vi "5.1-6.7.1-Act Client.vi"() -> ()   [LabVIEW 2010]
doc: "This VI implements a client for the Named Service UDP Server.vi.\nIt connects to a service by specifying the server address and the name of the service. After sending a 'Hello' string to the server, the client receives the string sent by the server, displays the string and closes the connection.\n\n<b>Note:</b> This VI is built to work with the Named Service UDP Server.vi in UDP.llb."
uses:
  6-OCU Neurons/MDF LatLong.ctl
  6-OCU Neurons/MDF Array LatLong.ctl
  6-OCU Neurons/6.1-UDP Saitek.ctl
  6-OCU Neurons/MainControls.ctl
  5.0-Global.vi
panel:
  out "data":T1 {"5.1.1 MDF GPS 2"."Latitude (waypoint)" format="%#_8g"; "5.1.1 MDF GPS 2"."Longitude  (waypoint)" format="%#_8g"; "6.1-Saitek Controller"."Right" scale=-32767.0..32767.0; "6.1-Saitek Controller"."Left" scale=-32767.0..32767.0; "6.1-Saitek Controller"."Yaw" scale=-32767.0..32767.0; "6.1-Saitek Controller"."Roll" scale=-32767.0..32767.0; "6.1-Saitek Controller"."Pitch" scale=-32767.0..32767.0}
  out "String":string
  out "error out":errorcluster
  in  "stop":bool
  in  "error in":errorcluster
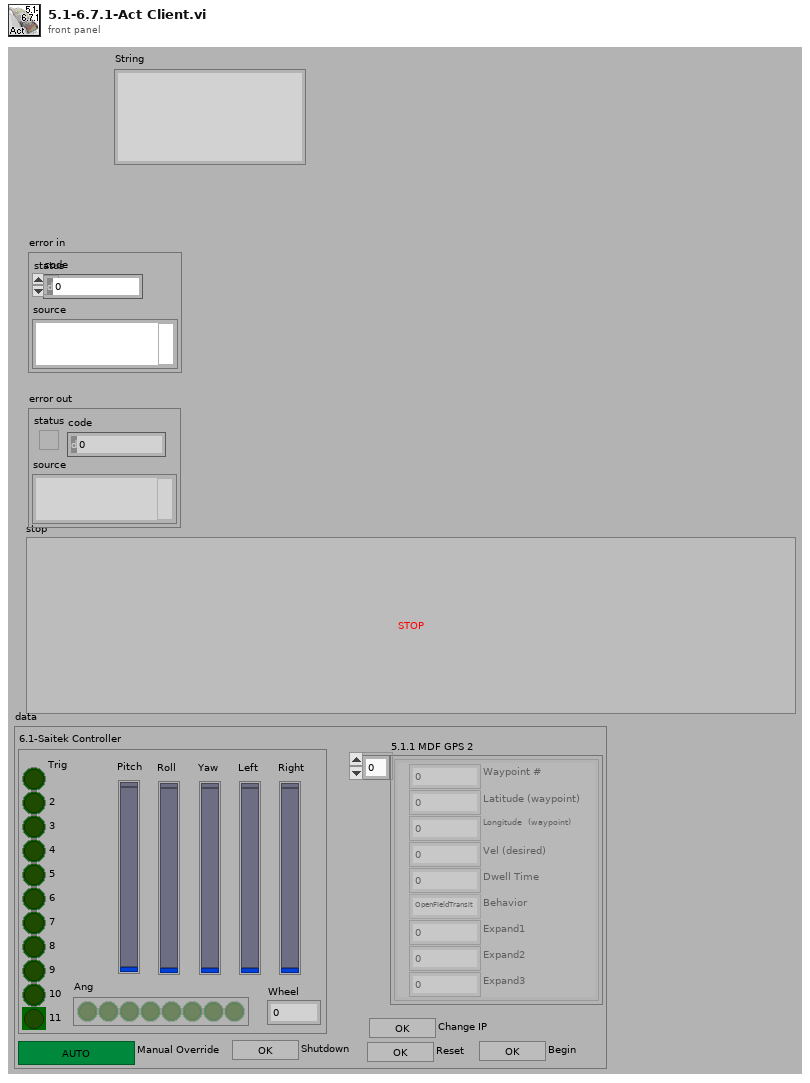
[diagram p1: front panel]
types:
  T1 = typedef "MainControls.ctl" = cluster{"6.1-Saitek Controller":T2, "Manual Override":bool, "5.1.1 MDF GPS 2":T3, "Shutdown":bool, "Reset":bool, "Change IP":bool, "Begin":bool}
  T2 = typedef "6.1-UDP Saitek.ctl" = cluster{"Trig":bool, "2":bool, "3":bool, "4":bool, "5":bool, "6":bool, "7":bool, "8":bool, "9":bool, "10":bool, "11":bool, "Pitch":i32, "Ang":bool[], "Wheel":dbl, "Roll":i32, "Yaw":i32, "Left":i32, "Right":i32}
  T3 = typedef "MDF Array LatLong.ctl" = T4[]
  T4 = typedef "MDF LatLong.ctl" = cluster{"Waypoint #":dbl, "Latitude (waypoint)":ext, "Longitude  (waypoint)":ext, "Vel (desired)":dbl, "Dwell Time":dbl, "Behavior":enum16{"OpenFieldTransit", "WallFollow", "LaneFollow", "ManualMode"}, "Expand1":dbl, "Expand2":dbl, "Expand3":dbl}
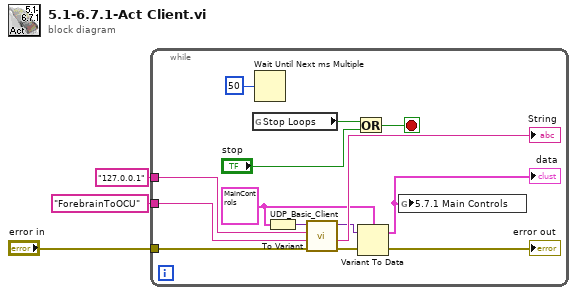
[diagram p0: block diagram]
diagram:
  n1 = while {
    tunnel: "ForebrainToOCU" -> [w11]
    tunnel: "error in" -> [w10]
    tunnel: "127.0.0.1" -> [w12]
    stop <- w16 stop-if-true
    w7 = T1 {"6.1-Saitek Controller"={"Trig"=FALSE, "2"=FALSE, "3"=FALSE, "4"=FALSE, "5"=FALSE, "6"=FALSE, "7"=FALSE, "8"=FALSE, "9"=FALSE, "10"=FALSE, "11"=FALSE, "Pitch"=0, "Ang"=[], "Wheel"=0.0, "Roll"=0, "Yaw"=0, "Left"=0, "Right"=0}, "Manual Override"=FALSE, "5.1.1 MDF GPS 2"=[], "Shutdown"=FALSE, "Reset"=FALSE, "Change IP"=FALSE, "Begin"=FALSE} ("Main Controls")
    n2 = global read "5.0-Global.vi" "Stop Loops"() -> (w15:bool)
    n3 = Wait Until Next ms Multiple(millisecond multiple=u32 50) -> ()  [unwired: 1 out]
    n4 = To Variant(anything=w7) -> (Variant=w13:variant)
    n5 = call "UDP_Basic_Client.vi"("error In"=w10, "Service Name"=w11, "IP Adress"=w12, "DataTypeIn"=w13) -> ("error IO"=w5:errorcluster, "String"=→"String":string, "DataOut"=w8:variant)  [unwired: 1 in]
    n6 = Or(x=w15, y="stop") -> (x .or. y?=w16:bool)
    n7 = Variant To Data(error in=w5, Variant=w8, type=w7) -> (error out=→"error out":errorcluster, data=w6:T1)
    "data" <- w6
    n8 = global write "5.0-Global.vi" "5.7.1 Main Controls"(w6) -> ()
  }
